vi "SubVI_runflag.vi"(7 "cmd":enum16{"write", "ini", "read"}(ring), 8 "error in (no error)":errorcluster caption="error in") -> (0 "error out":errorcluster, 3 "flag":bool)   [LabVIEW 2016]
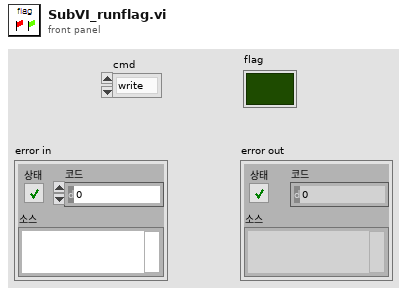
[diagram p1: front panel]
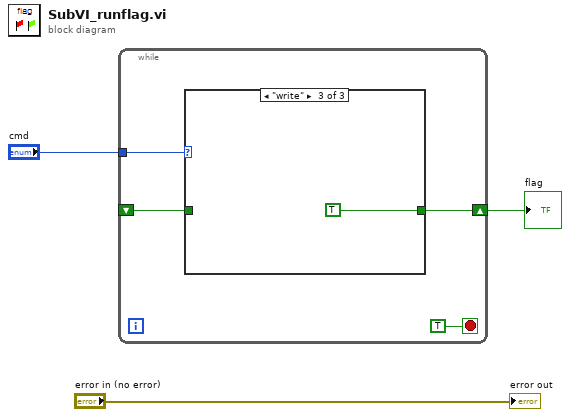
[diagram p0: block diagram]
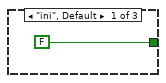
[diagram p2: hidden frame]
diagram:
  n1 = while {
    tunnel: "cmd" -> [w7]
    shift-right: [w5] -> w2
    shift-left: _ -> [w4]
    stop <- TRUE stop-if-true
    n2 = case shown="\"write\"" w7 {
      tunnel: [FALSE w9 TRUE ("value")] -> w5
      tunnel: w4 -> [_ w9 _]
      frame "ini", Default {
      }
      frame "read" {
      }
      frame "write" {
      }
    }
  }
  "flag" <- w2
  "error out" <- "error in (no error)"
